vi "formula node(1).vi"() -> ()   [LabVIEW 2013]
panel:
  out "output variable":dbl
  in  "m":dbl
  in  "x":dbl
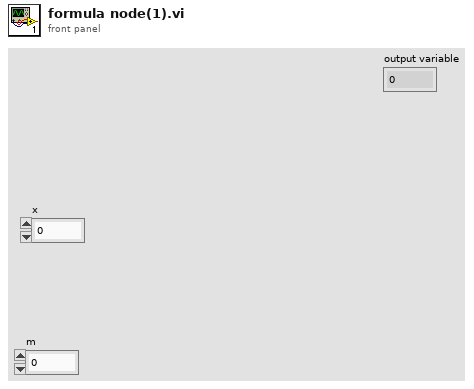
[diagram p1: front panel]
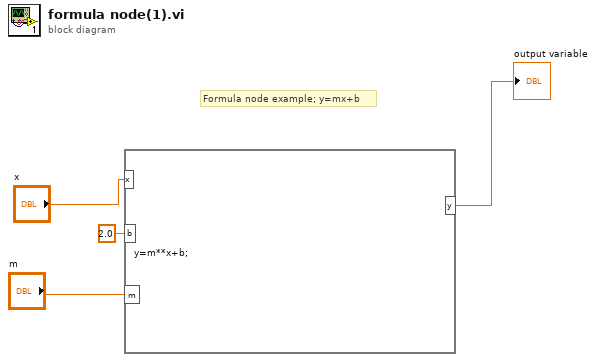
[diagram p0: block diagram]
diagram:
  # "Formula node example; y=mx+b"
  n1 = formula code="y=m**x+b;"("b"=2.0 ("input variable"), "x"="x", "m"="m") -> ("y"=→"output variable":dbl)
